vi "copySecvarChkresAndNoteFromIniToTable.vi"(8 "valInCol5":string, 9 "valInCol4":string, 10 "valInCol2":string, 11 "arrayAtSameRow":string[](array[string])) -> (3 "arrWithSecvar&Chkres&Note":string[](array[string]))   [LabVIEW 2010]
panel:
  # "secVar"
  # "chkRes"
  # "note"
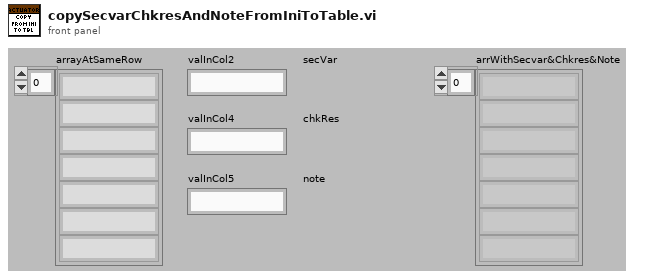
[diagram p1: front panel]
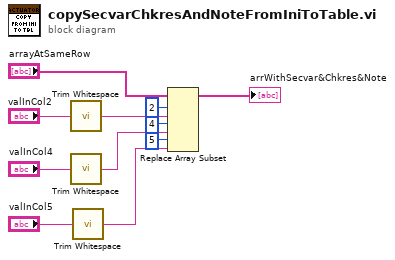
[diagram p0: block diagram]
diagram:
  n1 = call <vilib>:"Trim Whitespace.vi"("string"="valInCol2") -> ("trimmed string"=w5:string)  [unwired: 1 in]
  n2 = call <vilib>:"Trim Whitespace.vi"("string"="valInCol4") -> ("trimmed string"=w4:string)  [unwired: 1 in]
  n3 = call <vilib>:"Trim Whitespace.vi"("string"="valInCol5") -> ("trimmed string"=w3:string)  [unwired: 1 in]
  n4 = Replace Array Subset(array="arrayAtSameRow", new element #1=w5, index #1=2 ("index"), new element #2=w4, index #2=4 ("index"), new element #3=w3, index #3=5 ("index")) -> (→"arrWithSecvar&Chkres&Note":string[])
